vi "write_and_read.vi"(3 "error in":errorcluster, 4 "write buffer":string, 5 "VISA resource name in":refnum<visa-resource-name>) -> (0 "error out":errorcluster, 1 "read buffer":string, 2 "VISA resource name out":refnum<visa-resource-name>)   [LabVIEW 2016]
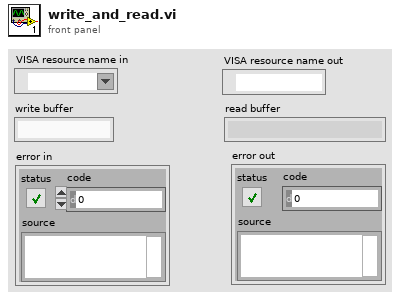
[diagram p1: front panel]
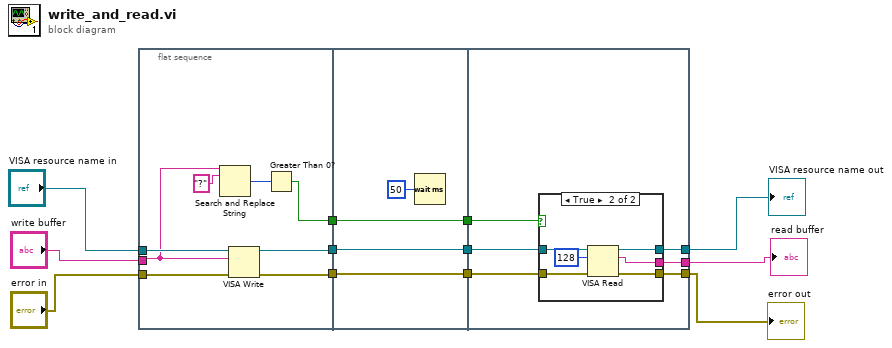
[diagram p0: block diagram]
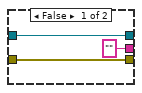
[diagram p2: hidden frame]
diagram:
  n1 = flat-sequence {
    tunnel: [w20] -> w12
    tunnel: [w19] -> w11
    tunnel: "VISA resource name in" -> [w18]
    tunnel: "error in" -> [w17]
    tunnel: "write buffer" -> [w16]
    tunnel: [w13] -> w1
    tunnel: w12 -> [w24]
    tunnel: [w24] -> w10
    tunnel: w11 -> [w23]
    tunnel: [w23] -> w9
    tunnel: [w21] -> w2
    tunnel: w1 -> [w21]
    tunnel: w10 -> [w30]
    tunnel: w9 -> [w29]
    tunnel: [w28] -> w6
    tunnel: [w27] -> w5
    tunnel: [w26] -> w3
    tunnel: w2 -> [w25]
    frame #0 {
      n2 = Search and Replace String(input string=w16, search string="?") -> (number of replacements=w14:i32)  [unwired: 6 in, 3 out]
      n3 = VISA Write(VISA resource name=w18, write buffer=w16, error in (no error)=w17) -> (VISA resource name out=w20:refnum<visa-resource-name>, error out=w19:errorcluster)  [unwired: 1 out]
      n4 = Greater Than 0?(x=w14) -> (x > 0?=w13:bool)
    }
    frame #1 {
      n5 = Wait (ms)(milliseconds to wait=u32 50) -> ()  [unwired: 1 out]
    }
    frame #2 {
      n6 = case shown="True" w25 {
        tunnel: w30 -> [w33 w38]
        tunnel: w29 -> [w32 w37]
        tunnel: [w33 w36] -> w28
        tunnel: [w32 w35] -> w27
        tunnel: ["" ("read buffer") w34] -> w26
        frame False {
        }
        frame True {
          n7 = VISA Read(VISA resource name=w38, byte count=u32 128, error in (no error)=w37) -> (VISA resource name out=w36:refnum<visa-resource-name>, read buffer=w34:string, error out=w35:errorcluster)  [unwired: 1 out]
        }
      }
    }
  }
  "VISA resource name out" <- w6
  "error out" <- w5
  "read buffer" <- w3
